vi "ScopeControl.vi"() -> ()   [LabVIEW 2011]
uses:
  <instrlib>/Tektronix TDS 3000 Series/Tektronix TDS 3000 Series.lvlib
panel:
  in  "error in (no error)":errorcluster {"code" format="%.0x"}
  in  "Save to Tree":bool
  in  "VISA Resource Name":refnum<visa-resource-name>="TCPIP0::10.10.10.41::INSTR"
  in  "?":T1(tab)
  in  "Channel 1 Enabled":bool=TRUE
  in  "Probe Attenuation 1":dbl=1.0 format="%.2f"
  in  "Channel Enabled":bool=TRUE
  in  "Probe Attenuation 2":dbl=1.0 format="%.2f"
  in  "Channel 3 Enabled":bool=TRUE
  in  "Probe Attenuation 3":dbl=1.0 format="%.2f"
  in  "Channel 4 Enabled":bool=TRUE
  in  "Probe Attenuation 4":dbl=1.0 format="%.2f"
  in  "Scale":dbl format="%.7f"
  in  "horiz pos 2":dbl format="%.7f"
  in  "horiz pos 1":dbl format="%.7f"
  in  "Scale":dbl format="%.7f"
  in  "vert pos 2":dbl format="%.7f"
  in  "vert pos 1":dbl format="%.7f"
  out "?":dbl[](graph)
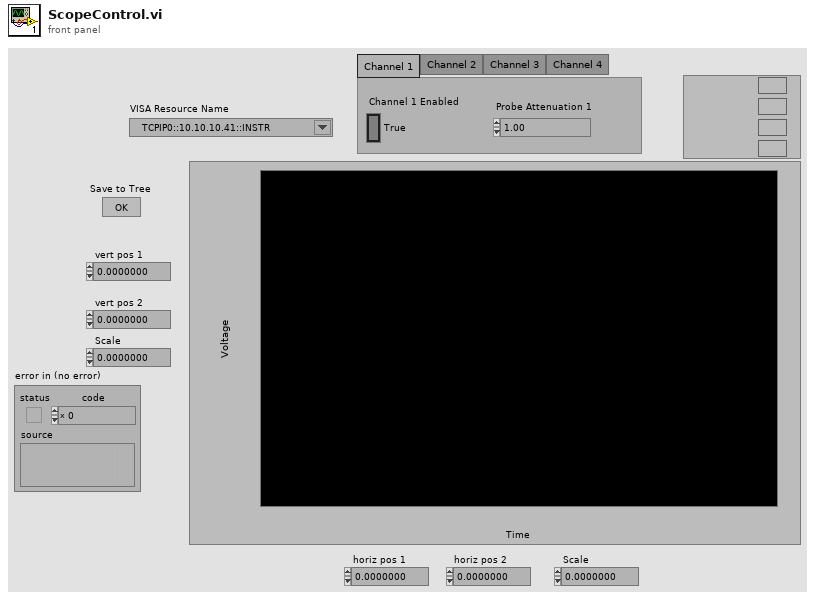
[diagram p1: front panel]
types:
  T1 = enum32{"Channel 1", "Channel 2", "Channel 3", "Channel 4"}
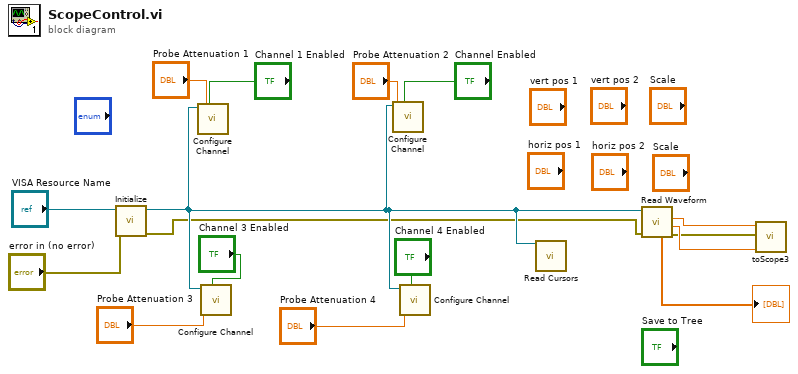
[diagram p0: block diagram]
diagram:
  n1 = call <instrlib>:"Initialize.vi"("error in (no error)"="error in (no error)", "VISA Resource Name"="VISA Resource Name") -> ("error out"=w1:errorcluster, "VISA Resource Name Out"=w6:refnum<visa-resource-name>)  [unwired: 8 in]
  n2 = call <instrlib>:"Configure Channel.vi"("Channel Enabled (True)"="Channel 1 Enabled", "Probe Attenuation (1.0)"="Probe Attenuation 1", "VISA Resource Name"=w6) -> ()  [unwired: 7 in, 2 out]
  n3 = call <instrlib>:"Configure Channel.vi"("Channel Enabled (True)"="Channel 3 Enabled", "Probe Attenuation (1.0)"="Probe Attenuation 3", "VISA Resource Name"=w6) -> ()  [unwired: 7 in, 2 out]
  n4 = call <instrlib>:"Configure Channel.vi"("Channel Enabled (True)"="Channel Enabled", "Probe Attenuation (1.0)"="Probe Attenuation 2", "VISA Resource Name"=w6) -> ()  [unwired: 7 in, 2 out]
  n5 = call <instrlib>:"Configure Channel.vi"("Channel Enabled (True)"="Channel 4 Enabled", "Probe Attenuation (1.0)"="Probe Attenuation 4", "VISA Resource Name"=w6) -> ()  [unwired: 7 in, 2 out]
  n6 = call <instrlib>:"Read Cursors.vi"("VISA Resource Name"=w6) -> ()  [unwired: 5 in, 10 out]
  n7 = call <instrlib>:"Read Waveform.vi"("error in (no error)"=w1, "VISA Resource Name"=w6) -> ("error out"=w3:errorcluster, "X Increment"=w5:dbl, "Initial X"=w4:dbl, "Waveform Array"=→"?":dbl[])  [unwired: 4 in, 2 out]
  n8 = call "toScope3.vi"("dt"=w5, "error in"=w3, "t0"=w4) -> ()  [unwired: 7 in, 2 out]
